vi "Msg.vi"(7 "Actor in":refnum<class "Actor.lvclass">, 11 "No Op Msg in":refnum<class "No Op Msg.lvclass">) -> (5 "Actor out":refnum<class "Actor.lvclass">)   [LabVIEW 2020, in "jettl.lvlib" / "No Op Msg.lvlib" / "No Op Msg.lvclass"]
uses:
  No Op Msg.lvclass
  Actor/Actor/Actor.lvclass
  No Op/No Op.lvclass
  No Op Msg.lvclass/No Op Msg.ctl
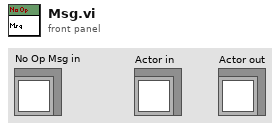
[diagram p1: front panel]
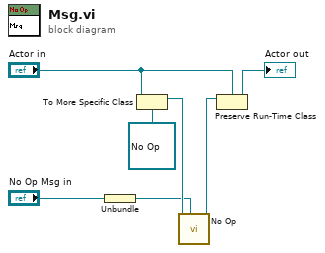
[diagram p0: block diagram]
diagram:
  n1 = Unbundle "Unbundle"("No Op Msg in") -> (w1:refnum<class "Sender.lvclass">)
  n2 = To More Specific Class(target class=refnum<class "No Op.lvclass"> refnum ("jettl.lvlib:No Op Msg.lvlib:No Op.lvclass"), reference="Actor in") -> (specific class reference=w3:refnum<class "No Op.lvclass">)  [unwired: 1 in, 1 out]
  n3 = call-dynamic "No Op.vi"("Sender"=w1, "No Op in"=w3) -> ("No Op out"=w2:refnum<class "No Op.lvclass">)  [unwired: 9 in]
  n4 = Preserve Run-Time Class(object in=w2, 2:"Actor in") -> (object out=→"Actor out":refnum<class "Actor.lvclass">)  [unwired: 1 in, 1 out]
